vi "ApplyQueuedMapUpdates.vi"(8 "error in (no error)":errorcluster, 11 "DirectedGraphWorldMap in":refnum<class "NI_Robotics_DirectedGraphWorldMap.lvclass">) -> (0 "error out":errorcluster, 3 "DirectedGraphWorldMap out":refnum<class "NI_Robotics_DirectedGraphWorldMap.lvclass">)   [LabVIEW 2017, in "NI_Robotics_DirectedGraphWorldMap.lvclass"]
uses:
  <vilib>/robotics/Navigation/shared/WorldMap/DirectedGraphWorldMap/NI_Robotics_DirectedGraphWorldMap.lvclass
  <vilib>/robotics/Navigation/shared/WorldMap/DirectedGraphWorldMap/NI_Robotics_DirectedGraphWorldMap.lvclass/NI_Robotics_DirectedGraphWorldMap.ctl
  <vilib>/robotics/Navigation/shared/MapNode/DirectedGraphMapNode/NI_Robotics_DirectedGraphMapNode.lvclass
  c:/Program Files (x86)/National Instruments/LabVIEW 2017/vi.lib/robotics/Navigation/shared/MapNode/AbstractDstarNode/NI_Robotics_AbstractDstarNode.lvclass
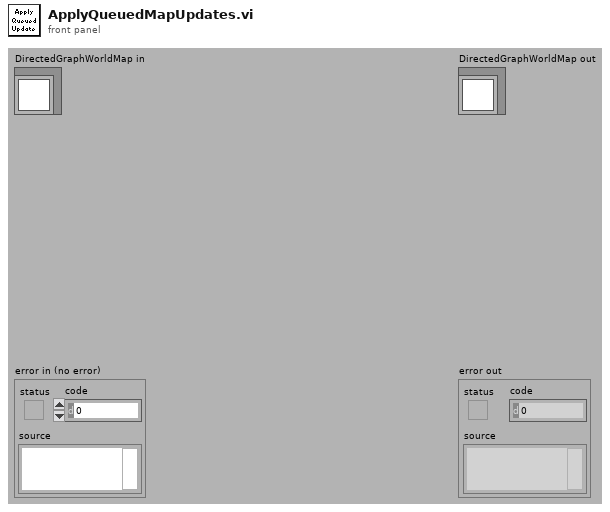
[diagram p1: front panel]
types:
  T1 = cluster{"Start":string, "End":string, "Cost":dbl}[]
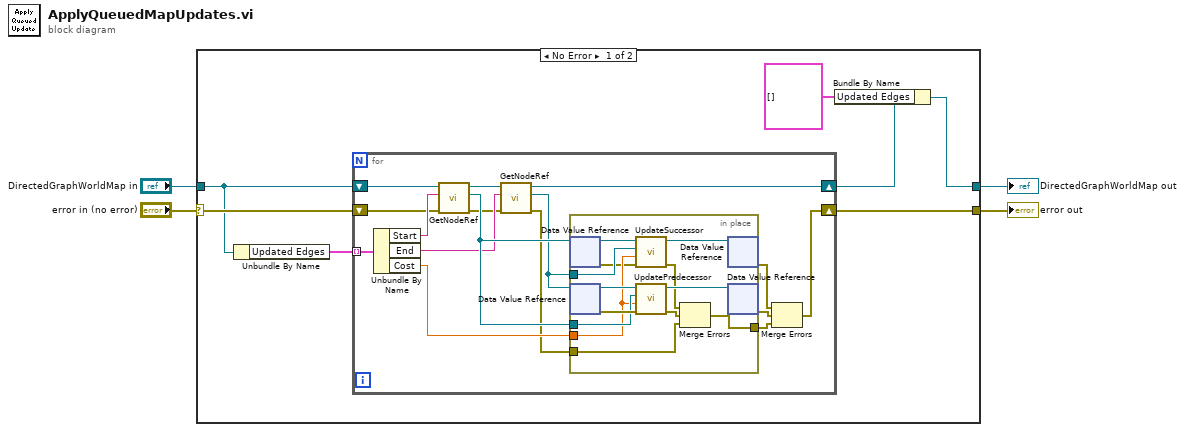
[diagram p0: block diagram]
diagram:
  n1 = case shown="No Error" "error in (no error)" {
    selector: "error in (no error)" -> [w9 w41]
    tunnel: "DirectedGraphWorldMap in" -> [w6 w42]
    tunnel: [w11 w42] -> w1
    tunnel: [w10 w41] -> w2
    frame No Error {
      n2 = Unbundle By Name(w6) -> ("Updated Edges"=w7:T1)
      n3 = for {
        tunnel: w7 -> [w27] mode=indexing
        shift-right: [w22] -> w10
        shift-left: w9 -> [w20]
        shift-right: [w12] -> w5
        shift-left: w6 -> [w13]
        n4 = Unbundle By Name(w27) -> ("Start"=w21:string, "End"=w16:string, "Cost"=w26:dbl)
        n5 = call <vilib>:"GetNodeRef.vi"("error in (no error)"=w20, "Node Name"=w21, "DirectedGraphWorldMap in"=w13) -> ("error out"=w15:errorcluster, "Node ref"=w19:refnum<data-value>, "DirectedGraphWorldMap out"=w18:refnum<class "NI_Robotics_DirectedGraphWorldMap.lvclass">)  [unwired: 5 in, 1 out]
        n6 = call <vilib>:"GetNodeRef.vi"("error in (no error)"=w15, "Node Name"=w16, "DirectedGraphWorldMap in"=w18) -> ("error out"=w14:errorcluster, "Node ref"=w17:refnum<data-value>, "DirectedGraphWorldMap out"=w12:refnum<class "NI_Robotics_DirectedGraphWorldMap.lvclass">)  [unwired: 5 in, 1 out]
        n7 = in-place {
          in-place-border: w26 -> [w34]
          in-place-border: w17 -> [w38]
          in-place-border: w19 -> [w35]
          in-place-border: [w32] -> w23
          in-place-border: w14 -> [w29]
          n8 = in-place-dvr #1(w19) -> (w40:refnum<class "NI_Robotics_DirectedGraphMapNode.lvclass">, w28:errorcluster)
          n9 = in-place-dvr #2(w17) -> (w37:refnum<class "NI_Robotics_DirectedGraphMapNode.lvclass">, w36:errorcluster)
          n10 = call-dynamic "UpdateSuccessor.vi"("error in (no error)"=w28, "Cost"=w34, "Successor Node Ref"=w38, "DirectedGraphMapNode in"=w40) -> ("error out"=w31:errorcluster, "DirectedGraphMapNode out"=w39:refnum<class "NI_Robotics_DirectedGraphMapNode.lvclass">)  [unwired: 6 in]
          n11 = call-dynamic "UpdatePredecessor.vi"("error in (no error)"=w36, "Cost"=w34, "Predecessor Node Ref"=w35, "DirectedGraphMapNode in"=w37) -> ("error out"=w30:errorcluster, "DirectedGraphMapNode out"=w33:refnum<class "NI_Robotics_DirectedGraphMapNode.lvclass">)  [unwired: 6 in]
          n12 = Merge Errors(w31, w30, w29) -> (w32:errorcluster)
          n13 = in-place-dvr #1(w39) -> (w25:errorcluster)  [unwired: 1 out]
          n14 = in-place-dvr #2(w33) -> (w24:errorcluster)  [unwired: 1 out]
        }
        n15 = Merge Errors(w25, w24, w23) -> (w22:errorcluster)
      }
      n16 = Bundle By Name(cluster=w5, "Updated Edges"=T1 []) -> (w11:refnum<class "NI_Robotics_DirectedGraphWorldMap.lvclass">)
    }
    frame Error {
    }
  }
  "error out" <- w2
  "DirectedGraphWorldMap out" <- w1
